vi "Main.vi"() -> ()   [LabVIEW 2020, in "Cloned UI.lvlib"]
uses:
  Cloned UI.lvlib
  Cloned Panel/Cloned Panel.lvclass
  C:/dev/LabVIEW/lv-oopanel/OOPanel/Panel/Panel.lvclass
  OOPanel/Manager/Manager.lvclass
panel:
  in  "Close All":bool
  in  "Hide All":bool
  in  "Show All":bool
  in  "New Clone":bool
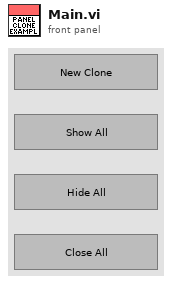
[diagram p1: front panel]
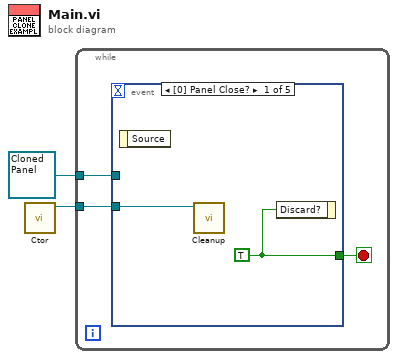
[diagram p0: block diagram]
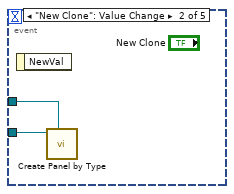
[diagram p2: hidden frame]
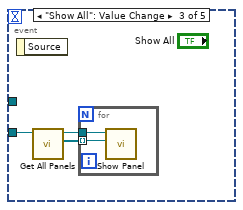
[diagram p3: hidden frame]
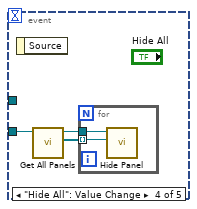
[diagram p4: hidden frame]
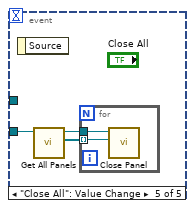
[diagram p5: hidden frame]
diagram:
  n1 = call "Ctor.vi"() -> ("Manager out"=w2:refnum<class "Manager.lvclass">)  [unwired: 10 in, 1 out]
  n2 = while {
    tunnel: w2 -> [w5]
    tunnel: refnum<class "Cloned Panel.lvclass"> refnum ("Cloned UI.lvlib:Cloned Panel.lvclass") -> [w3]
    stop <- w4 stop-if-true
    n3 = event shown="[0] Panel Close?" {
      selector: _ -> [_ _ _ _ _]
      dyn-events: _ -> [_ _ _ _ _]
      timeout: _ -> [_ _ _ _ _]
      tunnel: w5 -> [w7 w9 w12 w17 w22]
      tunnel: [w6 _ _ _ _] -> w4
      tunnel: w3 -> [_ w8 _ _ _]
      event Panel Close? {
        w6 = TRUE
        n4 = event-data() -> ()  [unwired: 1 in, 1 out]
        n5 = call "Cleanup.vi"("Manager in"=w7) -> ()  [unwired: 10 in, 1 out]
        n6 = event-data("Discard?"=w6) -> ()  [unwired: 1 in, 1 out]
      }
      event "New Clone": Value Change {
        n7 = event-data() -> ()  [unwired: 1 in, 1 out]
        n8 = call "Create Panel by Type.vi"("Panel Type"=w8, "Manager in"=w9) -> ()  [unwired: 7 in, 3 out]
      }
      event "Show All": Value Change {
        n9 = event-data() -> ()  [unwired: 1 in, 1 out]
        n10 = call "Get All Panels.vi"("Manager in"=w12) -> ("Panels"=w10:refnum<class "Panel.lvclass">[], "Manager out"=w11:refnum<class "Manager.lvclass">)  [unwired: 8 in, 1 out]
        n11 = for {
          tunnel: w11 -> [w14]
          tunnel: w10 -> [w13] mode=indexing
          n12 = call "Show Panel.vi"("Panel In"=w13, "Manager in"=w14) -> ()  [unwired: 7 in, 3 out]
        }
      }
      event "Hide All": Value Change {
        n13 = event-data() -> ()  [unwired: 1 in, 1 out]
        n14 = call "Get All Panels.vi"("Manager in"=w17) -> ("Panels"=w15:refnum<class "Panel.lvclass">[], "Manager out"=w16:refnum<class "Manager.lvclass">)  [unwired: 8 in, 1 out]
        n15 = for {
          tunnel: w16 -> [w19]
          tunnel: w15 -> [w18] mode=indexing
          n16 = call "Hide Panel.vi"("Panel In"=w18, "Manager in"=w19) -> ()  [unwired: 7 in, 3 out]
        }
      }
      event "Close All": Value Change {
        n17 = event-data() -> ()  [unwired: 1 in, 1 out]
        n18 = call "Get All Panels.vi"("Manager in"=w22) -> ("Panels"=w20:refnum<class "Panel.lvclass">[], "Manager out"=w21:refnum<class "Manager.lvclass">)  [unwired: 8 in, 1 out]
        n19 = for {
          tunnel: w21 -> [w24]
          tunnel: w20 -> [w23] mode=indexing
          n20 = call "Close Panel.vi"("Panel"=w23, "Manager in"=w24) -> ()  [unwired: 8 in, 2 out]
        }
      }
    }
  }
